vi "Get BPG Voltage.vi"(8 "error in (no error)":errorcluster, 10 "BPG Voltage":waveform(dbl)[](array[waveform]), 11 "BPG in":refnum<class "BPG.lvclass">) -> (0 "error out":errorcluster, 3 "BPG out":refnum<class "BPG.lvclass">)   [LabVIEW 2021, in "BPG.lvlib" / "BPG.lvclass"]
uses:
  BPG.lvclass
  BPG.lvclass/BPG.ctl
  <vilib>/ActorFramework/Actor/Actor.lvclass
  BPG Pressure/BPG Pressure Messages/BPG Pressure Msg/BPG Pressure Msg.lvclass
  <vilib>/Analysis/NI_AALBase.lvlib
  <vilib>/Analysis/baseanly.llb/Mean (DBL).vi
  <vilib>/NathanCo/Analog-Tasks/Analog Input/Analog Input/Analog Input/Analog Input.lvclass
  C:/Program Files/National Instruments/LabVIEW 2021/vi.lib/MGI/Panel Manager/Panel Actor/Panel Actor/Panel Actor.lvclass
  C:/Program Files/National Instruments/LabVIEW 2021/vi.lib/ActorFramework/Actor/Actor.lvclass
  C:/git/Pressure-Gauges/Files-to-be-organized/BPG/BPG/BPG.lvclass
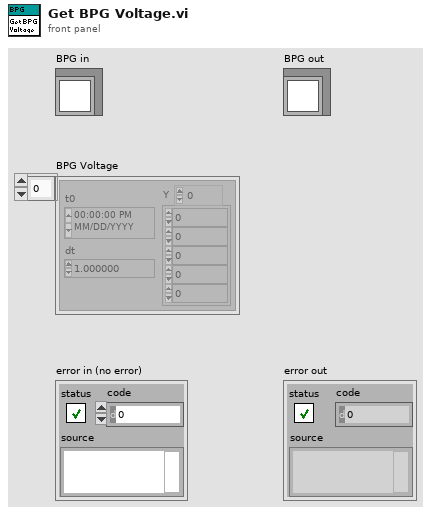
[diagram p1: front panel]
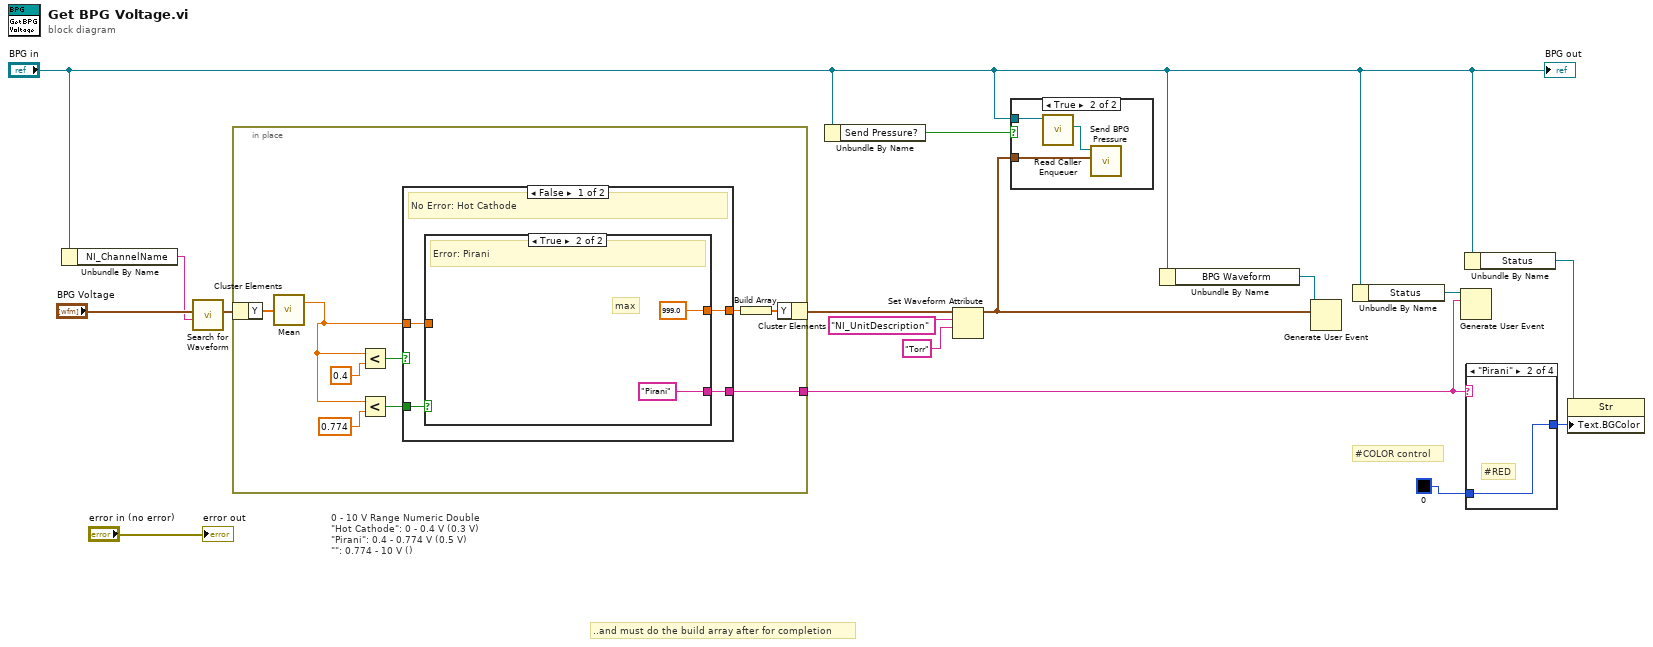
[diagram p0: block diagram]
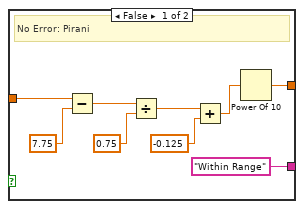
[diagram p6: hidden frame]
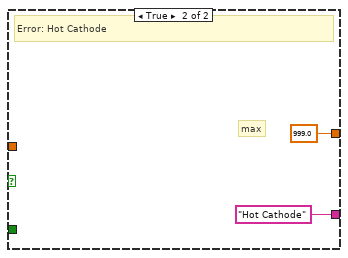
[diagram p7: hidden frame]
diagram:
  # "#COLOR control"
  # "..and must do the build array after for completion"
  # "0 - 10 V Range Numeric Double\n\"Hot Cathode\": 0 - 0.4 V (0.3 V)\n\"Pirani\": 0.4 - 0.774 V (0.5 V)\n\"\": 0.774 - 10 V ()"
  n1 = Unbundle By Name("BPG in") -> ("NI_ChannelName"=w1:string)
  n2 = call <vilib>:"Search for Waveform.vi"("NI_ChannelName"=w1, "Waveforms"="BPG Voltage") -> ("Waveform"=w3:waveform(dbl))  [unwired: 8 in, 1 out]
  n3 = in-place {
    in-place-border: [w25] -> w12
    n4 = in-place-cluster #1(w3) -> ("Y"=w18:dbl[])
    n5 = call-poly <vilib>:"Mean.vi"("X"=w18) -> ("mean"=w17:dbl)  [unwired: 1 out]
    n6 = Less?(x=w17, y=0.4) -> (x < y?=w22:bool)
    n7 = Less?(x=w17, y=0.774) -> (x < y?=w23:bool)
    n8 = case shown="False" w22 {
      tunnel: w23 -> [w29 _]
      tunnel: [w28 999.0] -> w24
      tunnel: w17 -> [w27 _]
      tunnel: [w26 "Hot Cathode"] -> w25
      frame False {
        # "No Error: Hot Cathode"
        n9 = case shown="True" w29 {
          tunnel: [w38 999.0] -> w28
          tunnel: w27 -> [w37 _]
          tunnel: ["Within Range" "Pirani"] -> w26
          frame False {
            # "No Error: Pirani"
            n10 = Subtract(x=w37, y=7.75) -> (x-y=w35:dbl)
            n11 = Divide(x=w35, y=0.75) -> (x/y=w33:dbl)
            n12 = Add(x=w33, y=-0.125) -> (x+y=w31:dbl)
            n13 = Power Of 10(x=w31) -> (10^x=w38:dbl)
          }
          frame True {
            # "max"
            # "Error: Pirani"
          }
        }
      }
      frame True {
        # "max"
        # "Error: Hot Cathode"
      }
    }
    n14 = Build Array(w24) -> (w19:dbl[])
    n15 = in-place-cluster #1("Y"=w19) -> (w7:waveform(dbl))
  }
  n16 = Unbundle By Name("BPG in") -> ("Send Pressure?"=w11:bool)
  n17 = Set Waveform Attribute(5:"Torr" ("name"), 6:"NI_UnitDescription" ("name"), 7:w7) -> (3:w6:waveform(dbl))  [unwired: 1 in, 2 out]
  n18 = case shown="True" w11 {
    tunnel: "BPG in" -> [_ w45]
    tunnel: w6 -> [_ w43]
    frame False {
    }
    frame True {
      n19 = call <vilib>:"Read Caller Enqueuer.vi"("Actor"=w45) -> ("Caller Enqueuer"=w44:refnum<class "Message Enqueuer.lvclass">)  [unwired: 10 in]
      n20 = call "Send BPG Pressure.vi"("BPG Pressure"=w43, "Message Enqueuer"=w44) -> ()  [unwired: 8 in, 2 out]
    }
  }
  n21 = Unbundle By Name("BPG in") -> ("BPG Waveform"=w15:refnum<user-event>)
  n22 = Generate User Event(user event=w15, event data cluster=w6) -> ()  [unwired: 2 in, 2 out]
  n23 = Unbundle By Name("BPG in") -> ("Status"=w14:refnum<user-event>)
  n24 = Generate User Event(user event=w14, event data cluster=w12) -> ()  [unwired: 2 in, 2 out]
  n25 = Unbundle By Name("BPG in") -> ("Status"=w13:refnum<vi>)
  n26 = case shown="\"Pirani\"" w12 {
    tunnel: [w46 w47 w48 w49] -> w5
    tunnel: u32 0 ("Text.Text Colors:BG Color") -> [w46 w47 w48 w49]
    frame "Hot Cathode" {
      # "#RED"
    }
    frame "Pirani" {
      # "#RED"
    }
    frame "Within Range" {
      # "#GREEN"
    }
    frame "Other", Default {
      # "#RED"
    }
  }
  n27 = property class="Str"(reference=w13, "Text.BGColor"=w5) -> ()  [unwired: 1 in, 2 out]
  "error out" <- "error in (no error)"
  "BPG out" <- "BPG in"
